vi "7.vi"() -> ()   [LabVIEW 2017]
panel:
  out "Array 2":dbl[](array[numeric])
  out "Decimal":u8
  in  "Ring":u16(ring) items=["Decimal", "Binary", "Octal", "Hexadecimal"]
  in  "Array":bool[](array[boolean])
  out "Octal":u8
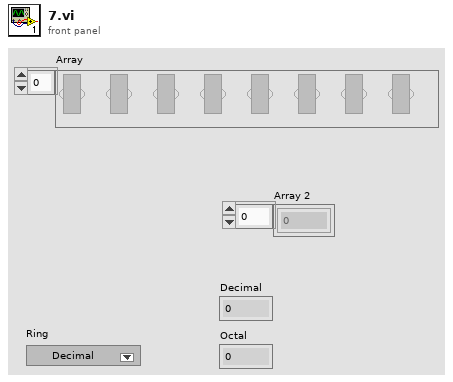
[diagram p1: front panel]
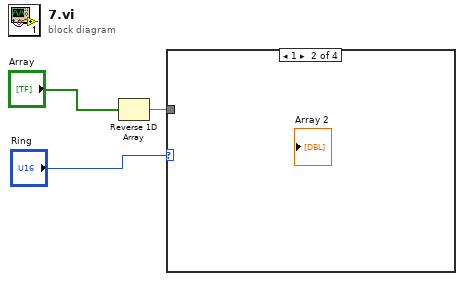
[diagram p0: block diagram]
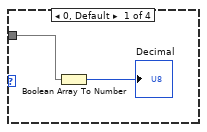
[diagram p2: hidden frame]
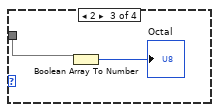
[diagram p3: hidden frame]
diagram:
  n1 = Reverse 1D Array(array="Array") -> (reversed array=w2:bool[])
  n2 = case shown="1" "Ring" {
    tunnel: w2 -> [w4 _ w6 _]
    frame 0, Default {
      n3 = Boolean Array To Number(Boolean array=w4) -> (number=→"Decimal":u32)
    }
    frame 1 {
    }
    frame 2 {
      n4 = Boolean Array To Number(Boolean array=w6) -> (number=→"Octal":u32)
    }
    frame 3 {
    }
  }
